vi "Main.vi"() -> ()   [LabVIEW 2017]
uses:
  Custom Controls/Heart Rate Parameters.ctl
  Custom Controls/State Control.ctl
panel:
  in  "Path for testing":path=path "BP DATA exp 2 116x77 63BPM.tdms"
  in  "Enable Automated Testing":bool
  out "error out":errorcluster
  in  "error in (no error)":errorcluster
  in  "Original Signal":dbl[](array[numeric])
  in  "Heart Rate Params":T1={"Heart Rates"=[], "Peak Pressures"=[], "Peak Amplitudes"=[], "History Length"=20, "Last  Slope"=20.0, "filtered history"=[], "raw history"=[], "Pulse"=FALSE, "Heart Rate Timer"=0, "Iteration"=0, "Pressure of Valley"=0.0, "Slope Log"=[], "Signal Segment"=refnum, "Acquisition Graph"=refnum, "This VI"=refnum, "Name"=""}
  out "Tab Control":enum32{"Test", "Results"}(tab)
  out "BPM":dbl format="%#.0f"
  in  "GO":bool
  out "Instant BPM":bool caption="Pulse"
  out "Signal Segment":dbl[](graph)
  in  "index":i32(slide)=15097 scale=0.0..30000.0
  in  "length":i32(slide)=25223 scale=0.0..60000.0
  out "Deviation":dbl(graph)=-0.00013401749999957245
  in  "Timming?":bool=TRUE
  out "Boolean":bool=TRUE
  out "Result Graph":cluster{"Pressure":dbl[], "Amplitude":dbl[]}(graph)={"Pressure"=[72.9592698, 75.39054775000001, 78.1595775, 80.79904660000001, 83.65028045, 86.62035345000001, 89.38759655, 92.79638935, 96.5009384, 100.08396834999999, 103.74116099999999, 107.97378269999999, 111.3575572, 115.57766925000001, 119.89785644999999, 124.36100744999999], "Amplitude"=[0.9122880000000038, 1.1410298500000096, 1.54758305, 1.8889093000000088, 2.0345532499999877, 2.061359100000004, 1.4877172499999887, 1.4734207500000025, 1.3992581499999943, 1.2857806999999895, 0.983769549999991, 1.2956095999999775, 0.8354451000000012, 0.627253550000006, 0.464632299999991, 0.4494424999999893, 0.0]}
  out "Systolic":dbl=113.56636759552792 format="%#.2f"
  out "Diastolic":dbl=77.06785498768801 format="%#.2f"
  out "Mean HR":dbl=62.36799130668109 format="%0.2f"
  out "name":string
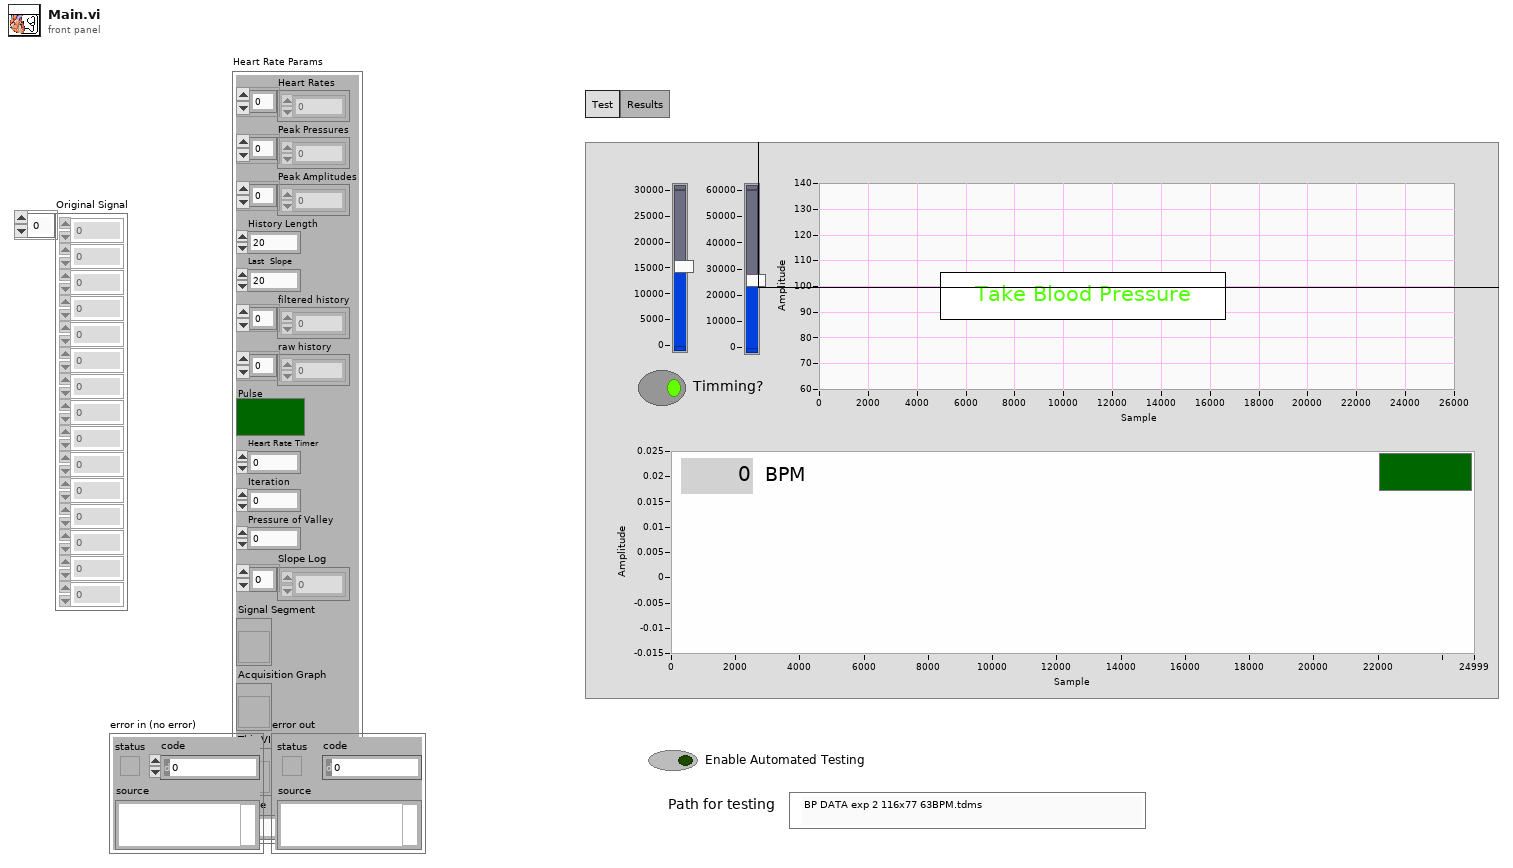
[diagram p1: front panel]
types:
  T1 = typedef "Heart Rate Parameters.ctl" = cluster{"Heart Rates":dbl[], "Peak Pressures":dbl[], "Peak Amplitudes":dbl[], "History Length":i32, "Last  Slope":dbl, "filtered history":dbl[], "raw history":dbl[], "Pulse":bool, "Heart Rate Timer":i32, "Iteration":u32, "Pressure of Valley":dbl, "Slope Log":dbl[], "Signal Segment":refnum<vi>, "Acquisition Graph":refnum<vi>, "This VI":refnum<vi>, "Name":string}
  T2 = typedef "State Control.ctl" = enum16{"Initialize", "Idle", "Inflate", "Abort", "Load Saved Data", "Set Display Window", "Analyze Input Data", "Calculate Pressure Values"}
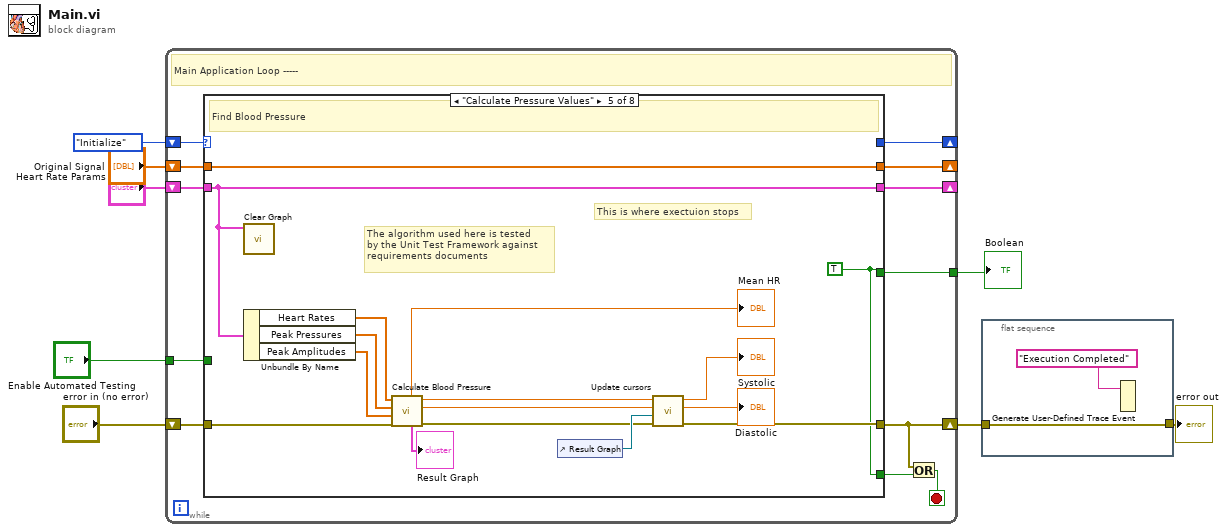
[diagram p0: block diagram]
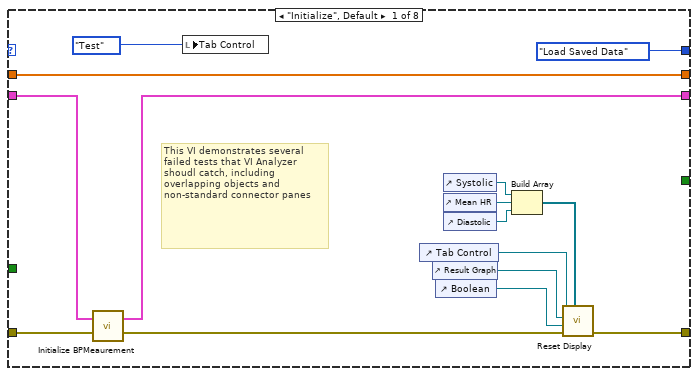
[diagram p2: hidden frame]
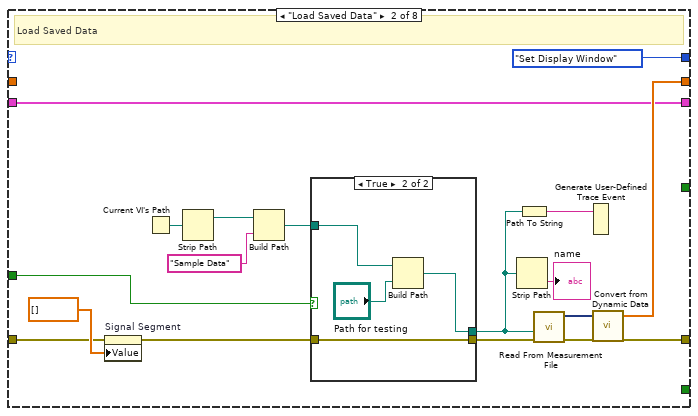
[diagram p3: hidden frame]
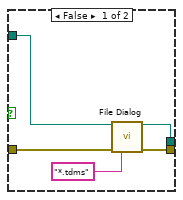
[diagram p4: hidden frame]
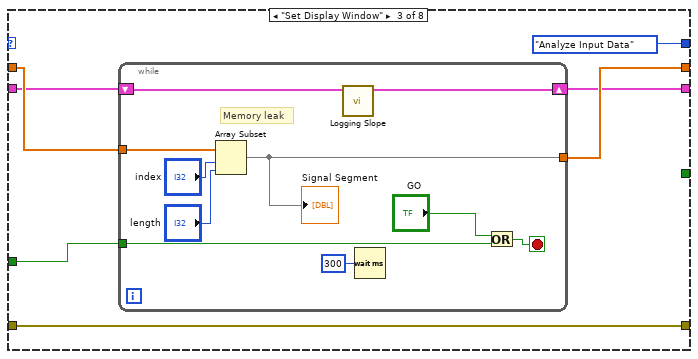
[diagram p5: hidden frame]
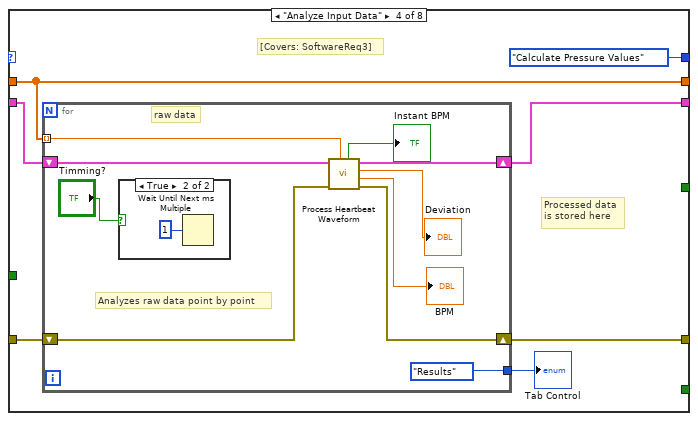
[diagram p6: hidden frame]
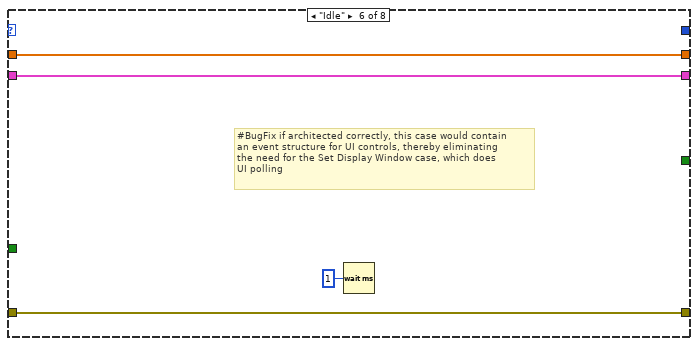
[diagram p8: hidden frame]
diagram:
  n1 = while {
    shift-right: [w10] -> w2
    shift-left: "error in (no error)" -> [w18]
    shift-right: [w17] -> _
    shift-left: State_Control."Initialize" ("State") -> [w19]
    shift-right: [w16] -> _
    shift-left: "Original Signal" -> [w15]
    shift-right: [w14] -> _
    shift-left: "Heart Rate Params" -> [w13]
    tunnel: "Enable Automated Testing" -> [w11]
    tunnel: [w9] -> w1
    stop <- w12 stop-if-true
    # "Main Application Loop -----"
    n2 = case shown="\"Calculate Pressure Values\"" w19 {
      tunnel: w18 -> [w23 w50 w63 w80 w108 w112 w118 w121]
      tunnel: [w28 w49 w63 w79 w101 w112 w118 w121] -> w10
      tunnel: [State_Control."Load Saved Data" ("State") State_Control."Set Display Window" ("State") State_Control."Analyze Input Data" ("State") State_Control."Calculate Pressure Values" ("State") _ _ _ _] -> w17
      tunnel: [w26 w48 w66 w81 w106 w115 w117 w120] -> w16
      tunnel: w15 -> [w26 _ w67 w81 w106 w115 w117 w120]
      tunnel: [w20 w46 w61 w83 w96 w113 w116 w119] -> w14
      tunnel: w13 -> [w25 w46 w62 w82 w96 w113 w116 w119]
      tunnel: w11 -> [_ w42 w64 _ _ _ _ _]
      tunnel: [_ _ _ _ w97 _ _ _] -> w9
      tunnel: [_ _ _ _ w97 _ _ _] -> w8
      frame "Initialize", Default {
        # "This VI demonstrates several failed tests that VI Analyzer shoudl catch, including overlapping objects and non-standard connector panes"
        n3 = call "Initialize BPMeaurement.vi"("error in (no error)"=w23, "Heart Rate Params"=w25) -> ("error out"=w22:errorcluster, "Heart Rate Params 2"=w20:T1)
        n4 = local write "Tab Control"(enum32{"Test", "Results"}."Test" ("Tab Control")) -> ()
        n5 = control-ref of="Tab Control"() -> (w24:refnum<vi>)
        n6 = control-ref of="Result Graph"() -> (w33:refnum<vi>)
        n7 = control-ref of="Boolean"() -> (w34:refnum<vi>)
        n8 = control-ref of="Systolic"() -> (w29:refnum<vi>)
        n9 = control-ref of="Mean HR"() -> (w31:refnum<vi>)
        n10 = control-ref of="Diastolic"() -> (w30:refnum<vi>)
        n11 = Build Array(w29, w31, w30) -> (w32:refnum<vi>[])
        n12 = call "Reset Display.vi"("Array"=w32, "error in (no error)"=w22, "Boolean"=w34, "Result Graph"=w33, "Tab Control"=w24) -> ("error out"=w28:errorcluster)  [unwired: 6 in]
      }
      frame "Load Saved Data" {
        # "Load Saved Data"
        n13 = property on="Signal Segment" class="WFGraph (strict)"(error in=w50, "Value"=dbl[] [] ("Signal Segment")) -> (error out=w45:errorcluster)  [unwired: 1 in, 1 out]
        n14 = Current VI's Path() -> (path=w41:path)
        n15 = Strip Path(path=w41) -> (stripped path=w37:path)  [unwired: 1 out]
        n16 = Build Path(base path=w37, name or relative path="Sample Data") -> (appended path=w39:path)
        n17 = case shown="True" w42 {
          tunnel: [w54 w58] -> w35
          tunnel: w45 -> [w56 w60]
          tunnel: [w55 w60] -> w44
          tunnel: w39 -> [w52 w59]
          frame False {
            n18 = call "File Dialog"("start path"=w52, "error in"=w56, "pattern (all files)"="*.tdms") -> ("selected path"=w54:path, "error out"=w55:errorcluster)  [unwired: 4 in, 7 out]
          }
          frame True {
            n19 = Build Path(base path=w59, name or relative path="Path for testing") -> (appended path=w58:path)
          }
        }
        n20 = Strip Path(path=w35) -> (name=→"name":string)  [unwired: 1 out]
        n21 = Path To String(path=w35) -> (string=w36:string)
        n22 = call "Read From Measurement File"("error in (no error)"=w44, "Filename"=w35) -> ("error out"=w49:errorcluster, "Signals"=w43:dynamicdata)  [unwired: 4 in, 4 out]
        n23 = Generate User-Defined Trace Event(2:w36) -> ()  [unwired: 1 in]
        n24 = call "Convert from Dynamic Data"("Dynamic Data Type"=w43) -> ("Array"=w48:dbl[])  [unwired: 3 out]
      }
      frame "Set Display Window" {
        n25 = while {
          tunnel: [w74] -> w66
          tunnel: w67 -> [w77]
          tunnel: w64 -> [w71]
          shift-right: [w68] -> w61
          shift-left: w62 -> [w69]
          stop <- w72 stop-if-true
          # "Memory leak"
          n26 = Array Subset(array=w77, index="index", length="length") -> (w74:dbl[])
          "Signal Segment" <- w74
          n27 = call "Logging Slope.vi"("Heart Rate Params"=w69) -> ("Heart Rate Params Out"=w68:T1)  [unwired: 8 in, 2 out]
          n28 = Wait (ms)(milliseconds to wait=u32 300) -> ()  [unwired: 1 out]
          n29 = Or(x="GO", y=w71) -> (x .or. y?=w72:bool)
        }
      }
      frame "Analyze Input Data" {
        # "Processed data\nis stored here"
        # "[Covers: SoftwareReq3]"
        n30 = for {
          shift-right: [w92] -> w83
          shift-left: w82 -> [w93]
          tunnel: [enum32{"Test", "Results"}."Results" ("Tab Control")] -> w84
          tunnel: w81 -> [w90] mode=indexing
          shift-right: [w86] -> w79
          shift-left: w80 -> [w87]
          # "raw data"
          # "Analyzes raw data point by point"
          n31 = case shown="True" "Timming?" {
            frame False {
            }
            frame True {
              n32 = Wait Until Next ms Multiple(millisecond multiple=u32 1) -> ()  [unwired: 1 out]
            }
          }
          n33 = call "Process Heartbeat Waveform.vi"("Pressure Measurement"=w90, "error in (no error)"=w87, "Heart Rate Params"=w93) -> ("error out"=w86:errorcluster, "BPM"=→"BPM":dbl, "Last Slope"=→"Deviation":dbl, "Heart Rate Params Out"=w92:T1, "Pulse"=→"Instant BPM":bool)  [unwired: 1 in, 3 out]
        }
        "Tab Control" <- w84
      }
      frame "Calculate Pressure Values" {
        w97 = TRUE
        # "This is where exectuion stops"
        # "The algorithm used here is tested \nby the Unit Test Framework against\nrequirements documents"
        # "Find Blood Pressure"
        n34 = call "Clear Graph.vi"("Heart Rate Params"=w96) -> ()  [unwired: 11 in]
        n35 = Unbundle By Name(w96) -> ("Heart Rates"=w110:dbl[], "Peak Pressures"=w111:dbl[], "Peak Amplitudes"=w109:dbl[])
        n36 = call "Calculate Blood Pressure.vi"("error in (no error)"=w108, "Peak Amplitudes"=w109, "Peak Pressures"=w111, "Heart Rates"=w110) -> ("error out"=w102:errorcluster, "Diastolic"=w104:dbl, "Systolic"=w105:dbl, "Output"=→"Result Graph":cluster{"Pressure":dbl[], "Amplitude":dbl[]}, "mean"=→"Mean HR":dbl)  [unwired: 3 in]
        n37 = control-ref of="Result Graph"() -> (w103:refnum<vi>)
        n38 = call "Update cursors.vi"("error in (no error)"=w102, "XY Graph Reference"=w103, "Diastolic IN"=w104, "Systolic IN"=w105) -> ("error Out"=w101:errorcluster, "Diastolic OUT"=→"Diastolic":dbl, "Systolic OUT"=→"Systolic":dbl)  [unwired: 5 in]
      }
      frame "Idle" {
        # "#BugFix if architected correctly, this case would contain\nan event structure for UI controls, thereby eliminating\nthe need for the Set Display Window case, which does\nUI polling"
        n39 = Wait (ms)(milliseconds to wait=u32 1) -> ()  [unwired: 1 out]
      }
      frame "Inflate" {
        # "#codeNeeded since this version of the code is designed\nto strictly simulate the algorithm, this\ncase has not been implemented. If used \nwith real hardware, it would be necessary to \ninflate the cuff first"
        # "[Covers: SoftwareReq3]"
      }
      frame "Abort" {
      }
    }
    n40 = Or(x=w10, y=w8) -> (x .or. y?=w12:bool)
  }
  "error out" <- w2
  "Boolean" <- w1
  n41 = flat-sequence {
    tunnel: [w122] -> _
    tunnel: w2 -> [w122]
    frame #0 {
      n42 = Generate User-Defined Trace Event(2:"Execution Completed" ("trace string")) -> ()  [unwired: 1 in]
    }
  }
